vi "Configure SPI Trigger.vi"(5 "Trigger Type (0: MOSI)":i32(ring) items=["MOSI", "MISO"], 6 "Pattern Width (2: 2)":i32(ring)=2 items=["1"=1, "2"=2, "3"=3, "4"=4, "5"=5, "6"=6, "7"=7, "8"=8, "9"=9, "10"=10, "11"=11, "12"=12, "13"=13, "14"=14, "15"=15, "16"=16, "17"=17, "18"=18, "19"=19, "20"=20], 7 "SPI Data (\"0x34XF\")":string="0x34XF", 8 "error in (no error)":errorcluster, 9 "Trigger State (0: Low)":i32(ring) items=["Low", "High"], 10 "Channel (1: Serial Bus 1)":i32(ring)=1 items=["Serial Bus 1"=1, "Serial Bus 2"=2, "Serial Bus 3"=3, "Serial Bus 4"=4], 11 "VISA resource name":refnum<visa-resource-name>) -> (0 "error out":errorcluster, 3 "VISA resource name out":refnum<visa-resource-name>)   [LabVIEW 2013, in "Agilent 90000 Series.lvlib"]
doc: "Configures SPI trigger settings.\n\n<B>Note:</B>\nYou must set decode mode to SPI using <B>Configure SBUS Normal.vi</B> before using this VI."
uses:
  Agilent 90000 Series.lvlib
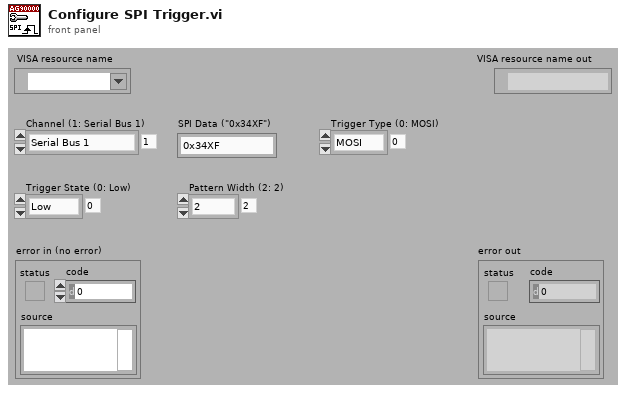
[diagram p1: front panel]
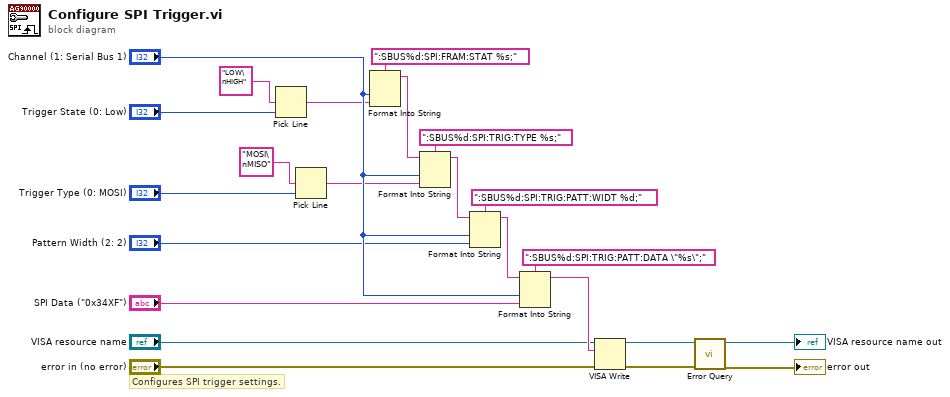
[diagram p0: block diagram]
diagram:
  # "Configures SPI trigger settings."
  n1 = Pick Line(multi-line string="LOW\nHIGH", line index="Trigger State (0: Low)") -> (output string=w19:string)  [unwired: 1 out]
  n2 = Pick Line(multi-line string="MOSI\nMISO", line index="Trigger Type (0: MOSI)") -> (output string=w14:string)  [unwired: 1 out]
  n3 = Format Into String(format string=":SBUS%d:SPI:FRAM:STAT %s;", "Channel (1: Serial Bus 1)", w19) -> (resulting string=w16:string)  [unwired: 2 in, 1 out]
  n4 = Format Into String(format string=":SBUS%d:SPI:TRIG:TYPE %s;", initial string=w16, "Channel (1: Serial Bus 1)", w14) -> (resulting string=w13:string)  [unwired: 1 in, 1 out]
  n5 = Format Into String(format string=":SBUS%d:SPI:TRIG:PATT:WIDT %d;", initial string=w13, "Channel (1: Serial Bus 1)", "Pattern Width (2: 2)") -> (resulting string=w10:string)  [unwired: 1 in, 1 out]
  n6 = Format Into String(format string=":SBUS%d:SPI:TRIG:PATT:DATA \"%s\";", initial string=w10, "Channel (1: Serial Bus 1)", "SPI Data (\"0x34XF\")") -> (resulting string=w7:string)  [unwired: 1 in, 1 out]
  n7 = VISA Write(VISA resource name="VISA resource name", write buffer=w7, error in (no error)="error in (no error)") -> (VISA resource name out=w4:refnum<visa-resource-name>, error out=w3:errorcluster)  [unwired: 1 out]
  n8 = call "Error Query.vi"("error in (no error)"=w3, "VISA resource name"=w4) -> ("error out"=→"error out":errorcluster, "VISA resource name out"=→"VISA resource name out":refnum<visa-resource-name>)  [unwired: 8 out]
